vi "Ask_delete.vi"   [LabVIEW 2022 SP3]
uses:
  Mic/Mic_Global.vi
panel:
  # "You have an empty test/insturment\n\nshoudl I remove the test/nstrument?"
types:
  T1 = typedef "PreferencesControl.ctl" = cluster{"Name of test":string, "Date":timestamp, "Location":string, "Template":string, "Soundcard":string, "resolution":u16, "Sampling rate":u16, "Ch1 Gain ":dbl, "Ch2 Gain":dbl, "Sample time (s)":dbl, "Pre-trigger (s)":dbl, "Hammer Threshold":dbl, "Positions":i16, "Taps/Position":i16, "Set Names":string, "Freq resolution":dbl, "Hammer cutoff":dbl, "Mic cutoff":dbl, "Double bounce ":dbl, "Hammer Cal":dbl, "dB Offset":dbl, "Accel Cal":dbl, "Vibrometer Cal":dbl, "Mic Cal":dbl, "Output":u16, "Voltage Cal":dbl, "Vibrometer Port":refnum<visa-resource-name>, "Range":u16, "High Pass":u16, "Bandwidth":u16, "X Range":cluster{"Minimum":dbl, "Maximum":dbl, "Increment":dbl, "Minor Increment":dbl, "Start":dbl}[], "Y Range":cluster{"Minimum":dbl, "Maximum":dbl, "Increment":dbl, "Minor Increment":dbl, "Start":dbl}[], "dB Spread":dbl, "Trigger":u16, "Ch_1":u8, "Ch_2":u8, "flip?":bool, "60Hz":bool, "Time offset":dbl, "Piezo Cal":dbl, "Default Notes":string}
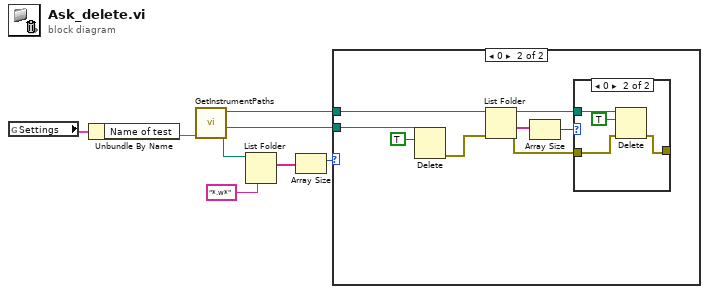
[diagram p0: block diagram]
diagram:
  n1 = global read "Mic_Global.vi" "Settings"() -> (w8:T1)
  n2 = Unbundle By Name(w8) -> ("Name of test"=w7:string)
  n3 = call "GetInstrumentPaths.vi"("Instrument"=w7) -> ("Path To Raw Folder"=w6:path, "Path To Test Folder"=w2:path, "Path To Instrument Folder"=w1:path)  [unwired: 6 in, 2 out]
  n4 = List Folder(path=w6, pattern="*.w*") -> (filenames=w4:string[])  [unwired: 2 in, 3 out]
  n5 = Array Size(array=w4) -> (size(s)=w3:i32)
  n6 = case shown="0" w3 {
    tunnel: w2 -> [_ w16]
    tunnel: w1 -> [_ w13]
    frame Default {
    }
    frame 0 {
      n7 = Delete(path (use dialog)=w16, entire hierarchy (F)=TRUE) -> (error out=w14:errorcluster)  [unwired: 3 in, 2 out]
      n8 = List Folder(path=w13, error in=w14) -> (path out=w10:path, folder names=w12:string[], error out=w9:errorcluster)  [unwired: 2 in, 1 out]
      n9 = Array Size(array=w12) -> (size(s)=w11:i32)
      n10 = case shown="0" w11 {
        tunnel: w10 -> [_ w19]
        tunnel: w9 -> [_ w18]
        tunnel: [_ w17] -> _
        frame Default {
        }
        frame 0 {
          n11 = Delete(path (use dialog)=w19, entire hierarchy (F)=TRUE, error in=w18) -> (error out=w17:errorcluster)  [unwired: 2 in, 2 out]
        }
      }
    }
  }
